vi "BNC555.evt call Config Sys (To) Trigger.vi"(0 "i ref in":refnum<vi>, 2 "Generator Instance":string="N/A", 3 "Mode":enum16{"Disabled", "Triggered", "Gated"}(ring), 4 "Trigger Level (2.5V)":dbl=2.5 format="%.4p", 5 "error in (no error)":errorcluster, 7 "Trigger Edge (T:Rising)":bool=TRUE, 9 "Gate Polarity (T:High)":bool=TRUE) -> (14 "i ref out":refnum<vi>, 19 "error out":errorcluster)   [LabVIEW 2014, in "BNC555.lvlib"]
doc: "This VI sends a simple event call to the wired BNC555."
uses:
  BNC555.lvlib
  CSCore/CSSystem/CoreLib/CoreLib.short 2 byte array.vi
  CSCore/CSSystem/CoreLib/CoreLib.double 2 byte array.vi
  CSCore/CSSystem/CoreLib/CoreLib.lvlib
  CSCore/BaseProcess/BaseProcess.lvlib
panel:
  # "High\nLow"
  # "Rising\nFalling"
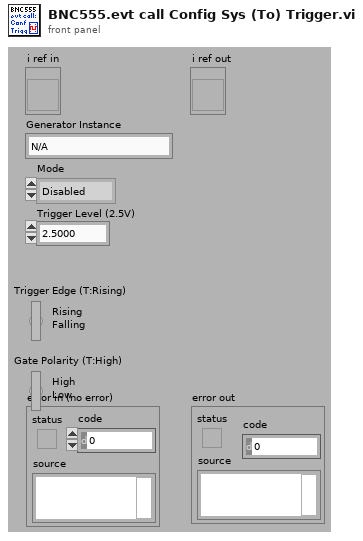
[diagram p1: front panel]
types:
  T1 = typedef "CoreDefs.rawDataType.ctl" = i8[]
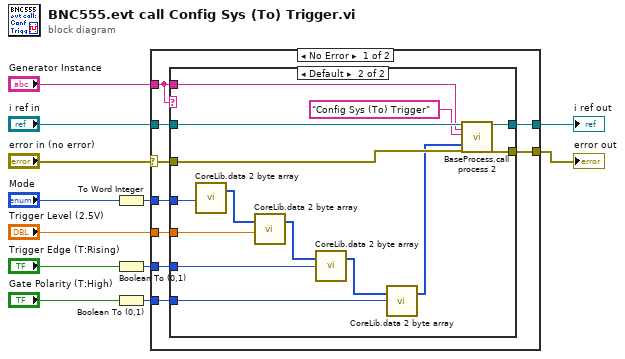
[diagram p0: block diagram]
diagram:
  n1 = To Word Integer(number="Mode") -> (16bit integer=w6:i16)
  n2 = Boolean To (0,1)(Boolean="Trigger Edge (T:Rising)") -> (0, 1=w3:i16)
  n3 = Boolean To (0,1)(Boolean="Gate Polarity (T:High)") -> (0, 1=w1:i16)
  n4 = case shown="No Error" "error in (no error)" {
    selector: "error in (no error)" -> [w18 w38]
    tunnel: [w21 w39] -> w11
    tunnel: [w20 w38] -> w10
    tunnel: "i ref in" -> [w19 w39]
    tunnel: "Generator Instance" -> [w17 _]
    tunnel: w6 -> [w16 _]
    tunnel: "Trigger Level (2.5V)" -> [w15 _]
    tunnel: w3 -> [w14 _]
    tunnel: w1 -> [w13 _]
    frame No Error {
      n5 = case shown="Default" w17 {
        tunnel: [w23 w37] -> w21
        tunnel: [w22 w36] -> w20
        tunnel: w19 -> [w23 w35]
        tunnel: w17 -> [_ w34]
        tunnel: w18 -> [w22 w32]
        tunnel: w16 -> [_ w27]
        tunnel: w15 -> [_ w26]
        tunnel: w14 -> [_ w25]
        tunnel: w13 -> [_ w24]
        frame "N/A" {
        }
        frame Default {
          n6 = call-poly "CoreLib.data 2 byte array.vi"("i16"=w27) -> ("byteArray out"=w31:T1)  [unwired: 18 in]
          n7 = call-poly "CoreLib.data 2 byte array.vi"("byteArray"=w31, "f64"=w26) -> ("byteArray out"=w30:T1)  [unwired: 17 in]
          n8 = call-poly "CoreLib.data 2 byte array.vi"("byteArray"=w30, "i16"=w25) -> ("byteArray out"=w29:T1)  [unwired: 17 in]
          n9 = call-poly "CoreLib.data 2 byte array.vi"("byteArray"=w29, "i16"=w24) -> ("byteArray out"=w28:T1)  [unwired: 17 in]
          n10 = call "BaseProcess.call process 2.vi"("i ref in"=w35, "Object"=w34, "Selector"="Config Sys (To) Trigger", "Data"=w28, "error in (no error)"=w32) -> ("i ref out"=w37:refnum<vi>, "error out"=w36:errorcluster)  [unwired: 13 in]
        }
      }
    }
    frame Error {
    }
  }
  "error out" <- w10
  "i ref out" <- w11
